vi "Host_Automate_Full_Timing_Study.vi"   [LabVIEW 2021]
types:
  T1 = cluster{"beam_length":dbl, "youngs_modulus":dbl, "torsion_spring":dbl, "beam_height":dbl, "beam_width":dbl, "beam_density":dbl, "number_of_FEA_nodes":i32, "accelerometer_mass":dbl}
  T2 = cluster{"Frequency KF":bool, "Pinned State KF":bool, "FFT Bounding":bool, "Filter Constants Frequency":cluster{"Measurement Variance":dbl, "State Variance":dbl, "Threshold":dbl}, "Filter Constants Position":cluster{"Measurement Variance":dbl, "State Variance":dbl, "Threshold":dbl}, "Moving Window Size":i32, "Time Series buffer":dbl, "Record Time Series Data":bool, "Record Moving Window Data":bool, "Record Online Error Metrics ":bool, "Record Statistics":bool}
  T3 = cluster{"Eigensolver ":enum16{"LabVIEW Cholesky", "LabVIEW General", "LabVIEW Inverse", "LEMP"}, "Models Forcasted":i32, "Max Roller Velocity":dbl, "Max Roller Position Percent":dbl, "Min Roller Position Percent":dbl}
  T4 = cluster{"Dataset":string, "Resample Method":enum16{"Recorded", "Auto Resample", "Custom Resample"}}
  T5 = cluster{"Modeling Parameters input controls":cluster{"beam_length":dbl, "youngs_modulus":dbl, "torsion_spring":dbl, "beam_height":dbl, "beam_width":dbl, "beam_density":dbl, "number_of_FEA_nodes":i32, "accelerometer_mass":dbl}, "Mockbear input controls":cluster{"Dataset":string, "Resample Method":enum16{"Recorded", "Auto Resample", "Custom Resample"}}, "Simulation Parameters input controls":cluster{"Eigensolver ":enum16{"LabVIEW Cholesky", "LabVIEW General", "LabVIEW Inverse", "LEMP"}, "Models Forcasted":i32, "Max Roller Velocity":dbl, "Max Roller Position Percent":dbl, "Min Roller Position Percent":dbl}, "Program Controls":cluster{"Frequency KF":bool, "Pinned State KF":bool, "FFT Bounding":bool, "Filter Constants Frequency":cluster{"Measurement Variance":dbl, "State Variance":dbl, "Threshold":dbl}, "Filter Constants Position":cluster{"Measurement Variance":dbl, "State Variance":dbl, "Threshold":dbl}, "Moving Window Size":i32, "Time Series buffer":dbl, "Record Time Series Data":bool, "Record Moving Window Data":bool, "Record Online Error Metrics ":bool, "Record Statistics":bool}}
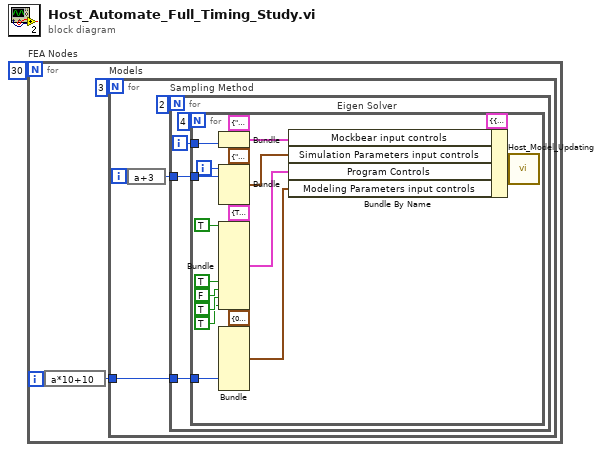
[diagram p0: block diagram]
diagram:
  n1 = for "FEA Nodes" {
    N: 30 -> [_]
    i -> [w3]
    n2 = expression code="a*10+10"(w3) -> (w2:i32)
    n3 = for "Models" {
      N: 3 -> [_]
      tunnel: w2 -> [w5]
      i -> [w7]
      n4 = expression code="a+3"(w7) -> (w6:i32)
      n5 = for "Sampling Method" {
        N: 2 -> [_]
        tunnel: w6 -> [w10]
        tunnel: w5 -> [w9]
        i -> [w11]
        n6 = for "Eigen Solver" {
          N: 4 -> [_]
          tunnel: w11 -> [w22]
          tunnel: w10 -> [w21]
          tunnel: w9 -> [w18]
          i -> [w23]
          n7 = Bundle(cluster=T4 {"Dataset"="test7", "Resample Method"=enum."Auto Resample"} ("Mockbear input controls"), "Resample Method"=w22) -> (w24:T4)  [unwired: 1 in]
          n8 = Bundle(cluster=T3 {"Eigensolver "=enum."LEMP", "Models Forcasted"=5, "Max Roller Velocity"=3.32, "Max Roller Position Percent"=0.43, "Min Roller Position Percent"=0.155} ("Simulation Parameters input controls"), "Eigensolver"=w23, "Models Forcasted"=w21) -> (w25:T3)  [unwired: 3 in]
          n9 = Bundle(cluster=T2 {"Frequency KF"=TRUE, "Pinned State KF"=FALSE, "FFT Bounding"=FALSE, "Filter Constants Frequency"={"Measurement Variance"=0.4, "State Variance"=0.01, "Threshold"=1000000000.0}, "Filter Constants Position"={"Measurement Variance"=0.4, "State Variance"=0.9, "Threshold"=1000000000.0}, "Moving Window Size"=10, "Time Series buffer"=10000.0, "Record Time Series Data"=FALSE, "Record Moving Window Data"=FALSE, "Record Online Error Metrics "=TRUE, "Record Statistics"=TRUE} ("Program Controls"), "Frequency KF"=TRUE, "Record Time Series Data"=TRUE, "Record Moving Window Data"=FALSE, "Record Online Error Metrics"=TRUE, "Record Statistics"=TRUE) -> (w30:T2)  [unwired: 6 in]
          n10 = Bundle(cluster=T1 {"beam_length"=0.3525, "youngs_modulus"=209500000000.0, "torsion_spring"=0.0, "beam_height"=0.00635, "beam_width"=0.0508, "beam_density"=7900.0, "number_of_FEA_nodes"=40, "accelerometer_mass"=0.055} ("Modeling Parameters input controls"), "number_of_FEA_nodes"=w18) -> (w19:T1)  [unwired: 7 in]
          n11 = Bundle By Name(cluster=T5 {"Modeling Parameters input controls"={"beam_length"=0.3525, "youngs_modulus"=209500000000.0, "torsion_spring"=0.0, "beam_height"=0.00635, "beam_width"=0.0508, "beam_density"=7900.0, "number_of_FEA_nodes"=40, "accelerometer_mass"=0.055}, "Mockbear input controls"={"Dataset"="test7", "Resample Method"=enum."Auto Resample"}, "Simulation Parameters input controls"={"Eigensolver "=enum."LEMP", "Models Forcasted"=5, "Max Roller Velocity"=3.32, "Max Roller Position Percent"=0.43, "Min Roller Position Percent"=0.155}, "Program Controls"={"Frequency KF"=TRUE, "Pinned State KF"=FALSE, "FFT Bounding"=FALSE, "Filter Constants Frequency"={"Measurement Variance"=0.4, "State Variance"=0.01, "Threshold"=1000000000.0}, "Filter Constants Position"={"Measurement Variance"=0.4, "State Variance"=0.9, "Threshold"=1000000000.0}, "Moving Window Size"=10, "Time Series buffer"=10000.0, "Record Time Series Data"=FALSE, "Record Moving Window Data"=FALSE, "Record Online Error Metrics "=TRUE, "Record Statistics"=TRUE}} ("Setup Parameters and Controls"), "Mockbear input controls"=w24, "Simulation Parameters input controls"=w25, "Program Controls"=w30, "Modeling Parameters input controls"=w19) -> (w31:T5)
          n12 = call "Host_Model_Updating.vi"("Setup Parameters and Controls"=w31) -> ()  [unwired: 11 in]
        }
      }
    }
  }
